vi "Label.vi"(11 "Numeric":i32) -> (3 "Array":dbl[][](array[numeric]))   [LabVIEW 2014]
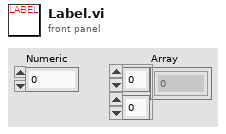
[diagram p1: front panel]
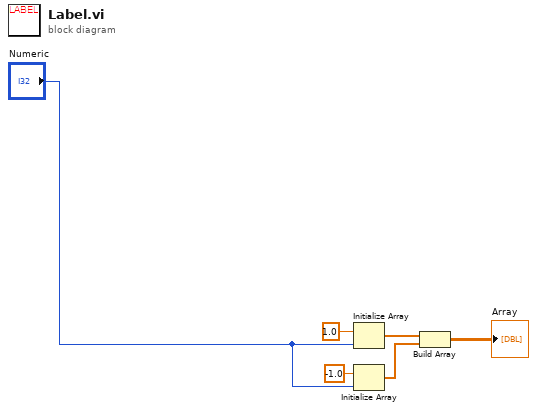
[diagram p0: block diagram]
diagram:
  n1 = Initialize Array(1.0 ("element"), "Numeric") -> (w4:dbl[])
  n2 = Initialize Array(-1.0 ("element"), "Numeric") -> (w5:dbl[])
  n3 = Build Array(w4, w5) -> (→"Array":dbl[][])
